vi "iWorx - Water Quality Lab.vi"() -> ()   [LabVIEW 2012]
uses:
  <vilib>/Utility/miscctls.llb/LVRangeTypeDef.ctl
  <vilib>/DAQmx/read.llb/DAQmx Read (Analog 1D Wfm NChan 1Samp).vi
  <vilib>/DAQmx/create/channels.llb/DAQmx Create Channel (AI-Voltage-Basic).vi
  <vilib>/DAQmx/miscellaneous.llb/DAQmx Fill In Error Info.vi
panel:
  in  "Mode":u16(ring) items=["Dissolved Oxygen", "pH", "Conductivity", "Turbidity"]
  in  "Set Up":bool
  out "Offset":dbl=-47.39336492890996
  out "Slope":dbl=47.39336492890995
  in  "Set SP2":bool
  in  "Set SP1":bool
  in  "Calibration Data":T1={"SP1 Voltage"=3.11, "SP2 Voltage"=1.0, "SP1 Value"=100.0, "SP2 Value"=0.0} {"SP2 Voltage" format="%#_g V"; "SP1 Voltage" format="%#_g V"}
  in  "Pause Button":bool
  in  "Snapshot":bool
  out "Processed Signal":dbl(knob) caption="Oxygen Content" scale=0.0..100.0
  in  "stop":bool
  out "Waveform Chart":waveform(dbl)(graph)
  in  "Sample Timing":u16(ring)=200 items=["20Hz"=50, "5 Hz"=200, "2 Hz"=500, "1 Hz"=1000, ".5 Hz"=2000, ".2 Hz"=5000]
  in  "Clear Chart":bool
  in  "Open Log":bool
  in  "Autoscale Y":bool
  out "Raw Signal":dbl(knob) scale=-5.0..5.0
  # "Water Quality Lab"
  # "Sensor Input (Ch 1)"
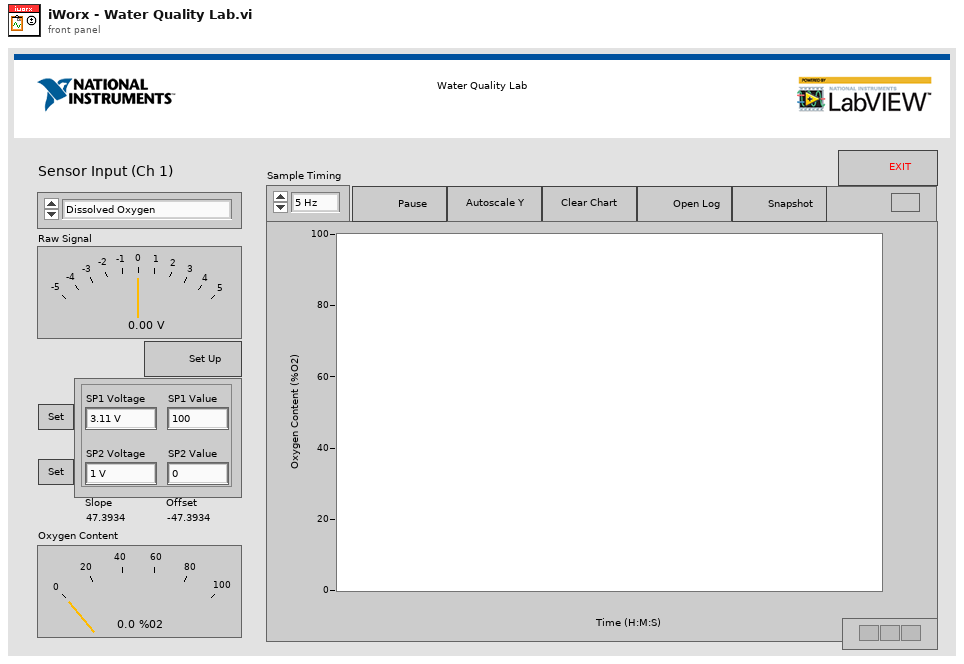
[diagram p1: front panel]
types:
  T1 = cluster{"SP1 Voltage":dbl, "SP2 Voltage":dbl, "SP1 Value":dbl, "SP2 Value":dbl}
  T2 = typedef "LVRangeTypeDef.ctl" = cluster{"Minimum":dbl, "Maximum":dbl, "Increment":dbl, "Minor Increment":dbl, "Start":dbl}
  T3 = cluster{"Name":string, "Format String":string, "Y Scale Name":string, "Scale.Range":T2, "Calibration Data":cluster{"SP1 Voltage":dbl, "SP2 Voltage":dbl, "SP1 Value":dbl, "SP2 Value":dbl}}[]
  T4 = cluster{"Name":string, "Format String":string, "Y Scale Name":string, "Scale.Range":T2, "Calibration Data":cluster{"SP1 Voltage":dbl, "SP2 Voltage":dbl, "SP1 Value":dbl, "SP2 Value":dbl}}
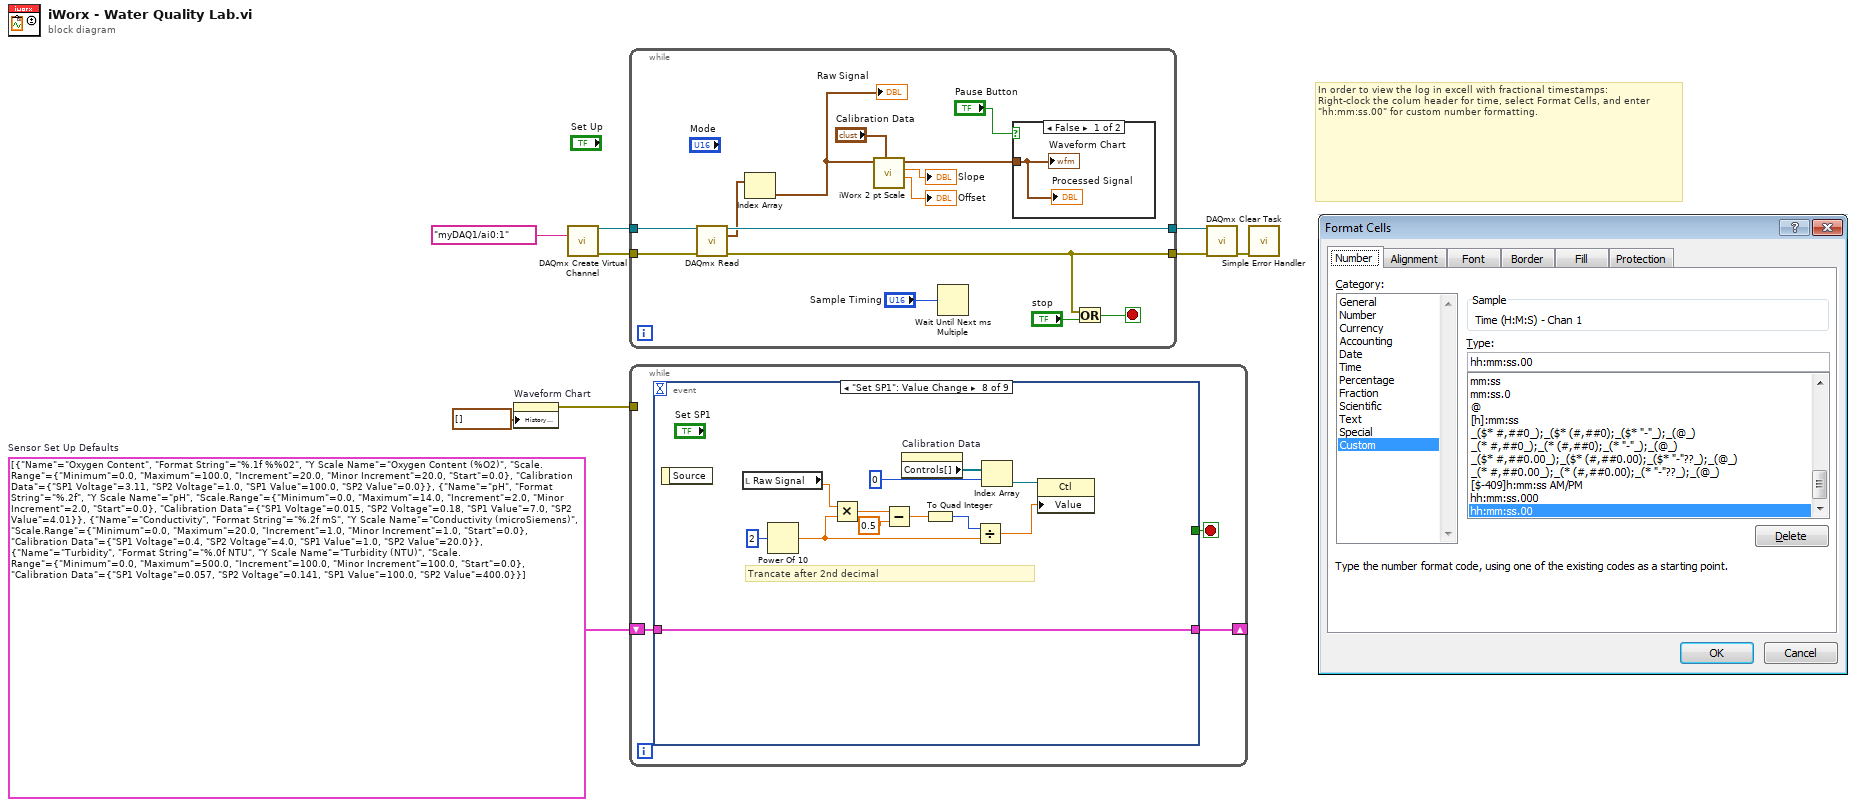
[diagram p0: block diagram]
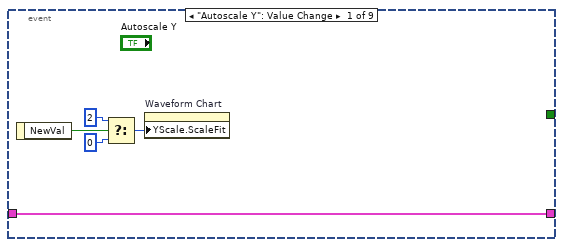
[diagram p2: hidden frame]
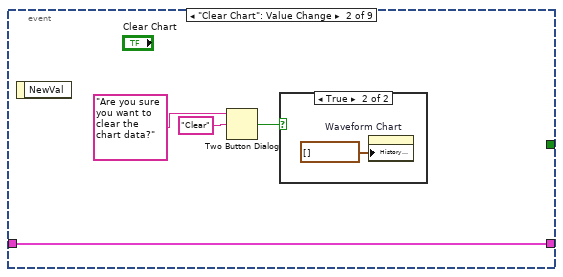
[diagram p3: hidden frame]
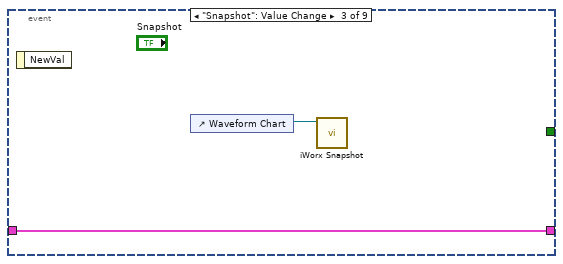
[diagram p5: hidden frame]
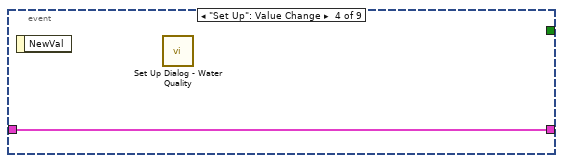
[diagram p6: hidden frame]
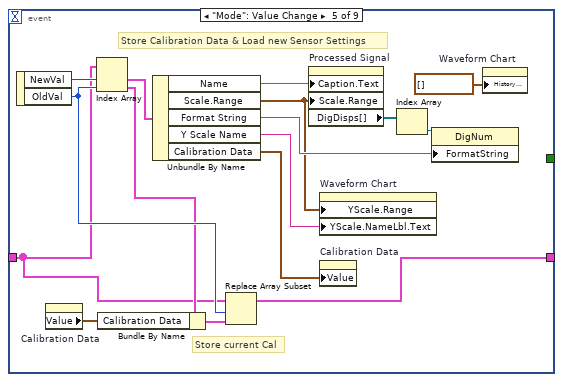
[diagram p7: hidden frame]
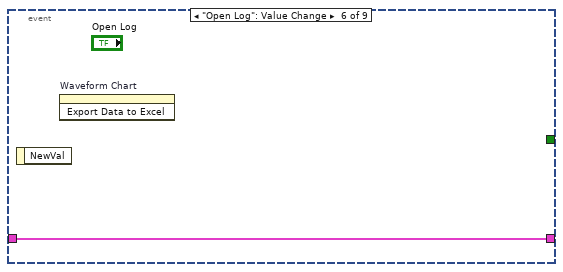
[diagram p8: hidden frame]
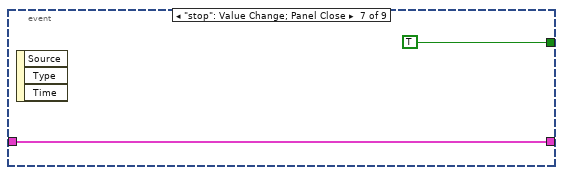
[diagram p9: hidden frame]
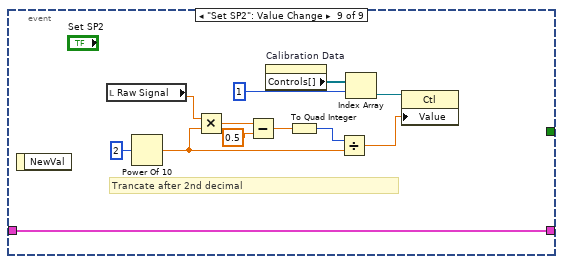
[diagram p10: hidden frame]
diagram:
  w1 = T3 [{"Name"="Oxygen Content", "Format String"="%.1f %%02", "Y Scale Name"="Oxygen Content (%O2)", "Scale.Range"={"Minimum"=0.0, "Maximum"=100.0, "Increment"=20.0, "Minor Increment"=20.0, "Start"=0.0}, "Calibration Data"={"SP1 Voltage"=3.11, "SP2 Voltage"=1.0, "SP1 Value"=100.0, "SP2 Value"=0.0}}, {"Name"="pH", "Format String"="%.2f", "Y Scale Name"="pH", "Scale.Range"={"Minimum"=0.0, "Maximum"=14.0, "Increment"=2.0, "Minor Increment"=2.0, "Start"=0.0}, "Calibration Data"={"SP1 Voltage"=0.015, "SP2 Voltage"=0.18, "SP1 Value"=7.0, "SP2 Value"=4.01}}, {"Name"="Conductivity", "Format String"="%.2f mS", "Y Scale Name"="Conductivity (microSiemens)", "Scale.Range"={"Minimum"=0.0, "Maximum"=20.0, "Increment"=1.0, "Minor Increment"=1.0, "Start"=0.0}, "Calibration Data"={"SP1 Voltage"=0.4, "SP2 Voltage"=4.0, "SP1 Value"=1.0, "SP2 Value"=20.0}}, {"Name"="Turbidity", "Format String"="%.0f NTU", "Y Scale Name"="Turbidity (NTU)", "Scale.Range"={"Minimum"=0.0, "Maximum"=500.0, "Increment"=100.0, "Minor Increment"=100.0, "Start"=0.0}, "Calibration Data"={"SP1 Voltage"=0.057, "SP2 Voltage"=0.141, "SP1 Value"=100.0, "SP2 Value"=400.0}}]  # Sensor Set Up Defaults
  # "In order to view the log in excell with fractional timestamps: \nRight-clock the colum header for time, select Format Cells, and enter \"hh:mm:ss.00\" for custom number formatting."
  n1 = property on="Waveform Chart" class="WFChart (strict)"("History Data"=waveform(dbl)[] []) -> (error out=w4:errorcluster)  [unwired: 2 in, 1 out]
  n2 = call-poly <vilib>:"DAQmx Create Virtual Channel.vi"("physical channels"=tag "myDAQ1/ai0:1") -> ("task out"=w6:refnum<k21>, "error out"=w5:errorcluster)  [unwired: 13 in]
  n3 = while {
    tunnel: w6 -> [w21]
    tunnel: [w20] -> w9
    tunnel: w5 -> [w19]
    tunnel: [w17] -> w8
    stop <- w18 stop-if-true
    n4 = call-poly <vilib>:"DAQmx Read.vi"("task/channels in"=w21, "error in"=w19) -> ("task out"=w20:refnum<k21>, "data"=w15:waveform(dbl)[], "error out"=w17:errorcluster)  [unwired: 11 in]
    n5 = Index Array(array=w15) -> (element=w13:waveform(dbl))  [unwired: 1 in]
    "Raw Signal" <- w13
    n6 = call "iWorx 2 pt Scale.vi"("Calibration Data"="Calibration Data", "Raw Waveform"=w13) -> ("Offset"=→"Offset":dbl, "Slope"=→"Slope":dbl, "Scaled Value"=w14:waveform(dbl))  [unwired: 7 in]
    n7 = Wait Until Next ms Multiple(millisecond multiple="Sample Timing") -> ()  [unwired: 1 out]
    n8 = case shown="False" "Pause Button" {
      tunnel: w14 -> [w24 _]
      frame False {
        "Waveform Chart" <- w24
        "Processed Signal" <- w24
      }
      frame True {
      }
    }
    n9 = Or(x=w17, y="stop") -> (x .or. y?=w18:bool)
  }
  n10 = while {
    tunnel: w4 -> [_]
    shift-right: [w25] -> _
    shift-left: w1 -> [w26]
    stop <- w27 stop-if-true
    n11 = event shown="[7] \"Set SP1\": Value Change" {
      selector: _ -> [_ _ _ _ _ _ _ _ _]
      dyn-events: _ -> [_ _ _ _ _ _ _ _ _]
      timeout: _ -> [_ _ _ _ _ _ _ _ _]
      tunnel: [_ _ _ _ _ _ TRUE _ _] -> w27
      tunnel: w26 -> [w28 w33 w38 w40 w41 w57 w58 w60 w72]
      tunnel: [w28 w33 w38 w40 w46 w57 w58 w60 w72] -> w25
      event "Autoscale Y": Value Change {
        n12 = event-data() -> ("NewVal"=w30:bool)  [unwired: 1 in]
        n13 = Select(t=u8 2 ("Y Scale.Scale Fit"), s=w30, f=u8 0 ("Y Scale.Scale Fit")) -> (s? t:f=w29:u8)
        n14 = property on="Waveform Chart" class="WFChart (strict)"("YScale.ScaleFit"=w29) -> ()  [unwired: 2 in, 2 out]
      }
      event "Clear Chart": Value Change {
        n15 = event-data() -> ()  [unwired: 1 in, 1 out]
        n16 = Two Button Dialog(message="Are you sure you want to clear the chart data?", 2:"Clear" ("T button name (\"OK\")")) -> (T button?=w35:bool)  [unwired: 1 in]
        n17 = case shown="True" w35 {
          frame False {
          }
          frame True {
            n18 = property on="Waveform Chart" class="WFChart (strict)"("History Data"=waveform(dbl)[] []) -> ()  [unwired: 2 in, 2 out]
          }
        }
      }
      event "Snapshot": Value Change {
        n19 = event-data() -> ()  [unwired: 1 in, 1 out]
        n20 = control-ref of="Waveform Chart"() -> (w39:refnum<vi>)
        n21 = call "iWorx Snapshot.vi"("WaveformChart in"=w39) -> ()  [unwired: 10 in, 1 out]
      }
      event "Set Up": Value Change {
        n22 = event-data() -> ()  [unwired: 1 in, 1 out]
        n23 = call "Set Up Dialog - Water Quality.vi"() -> ()  [unwired: 12 in]
      }
      event "Mode": Value Change {
        # "Store current Cal"
        # "Store Calibration Data & Load new Sensor Settings"
        n24 = event-data() -> ("NewVal"=w49:u16, "OldVal"=w47:u16)  [unwired: 1 in]
        n25 = property on="Calibration Data" class="Clust (strict)"() -> ("Value"=w45:T1)  [unwired: 2 in, 2 out]
        n26 = Index Array(array=w41, index #1=w49, index #2=w47) -> (element #1=w48:T4, element #2=w42:T4)
        n27 = Bundle By Name(cluster=w42, "Calibration Data"=w45) -> (w44:T4)
        n28 = Unbundle By Name(w48) -> ("Name"=w54:string, "Scale.Range"=w52:T2, "Format String"=w53:string, "Y Scale Name"=w51:string, "Calibration Data"=w50:T1)
        n29 = Replace Array Subset(array=w41, new element=w44, index=w47) -> (w46:T3)
        n30 = property on="Processed Signal" class="Knob (strict)"("Caption.Text"=w54, "Scale.Range"=w52) -> ("DigDisps[]"=w55:refnum<vi>[])  [unwired: 2 in, 2 out]
        n31 = property on="Waveform Chart" class="WFChart (strict)"("YScale.Range"=w52, "YScale.NameLbl.Text"=w51) -> ()  [unwired: 2 in, 2 out]
        n32 = property on="Calibration Data" class="Clust (strict)"("Value"=w50) -> ()  [unwired: 2 in, 2 out]
        n33 = Index Array(array=w55) -> (element=w56:refnum<vi>)  [unwired: 1 in]
        n34 = property class="DigNum"(reference=w56, "FormatString"=w53) -> ()  [unwired: 1 in, 2 out]
        n35 = property on="Waveform Chart" class="WFChart (strict)"("History Data"=waveform(dbl)[] []) -> ()  [unwired: 2 in, 2 out]
      }
      event "Open Log": Value Change {
        n36 = event-data() -> ()  [unwired: 1 in, 1 out]
        n37 = invoke on="Waveform Chart" class="WFChart (strict)" method="Export Data to Excel"() -> ()  [unwired: 3 in, 3 out]
      }
      event "stop": Value Change; Panel Close {
        n38 = event-data() -> ()  [unwired: 1 in, 3 out]
      }
      event "Set SP1": Value Change {
        # "Trancate after 2nd decimal"
        n39 = event-data() -> ()  [unwired: 1 in, 1 out]
        n40 = local read "Raw Signal"() -> (w61:dbl)
        n41 = Power Of 10(x=2) -> (10^x=w68:dbl)
        n42 = Multiply(x=w61, y=w68) -> (x*y=w66:dbl)
        n43 = Subtract(x=w66, y=0.5) -> (x-y=w65:dbl)
        n44 = property on="Calibration Data" class="Clust (strict)"() -> ("Controls[]"=w71:refnum<vi>[])  [unwired: 2 in, 2 out]
        n45 = To Quad Integer(1:w65) -> (0:w67:i64)
        n46 = Divide(x=w67, y=w68) -> (x/y=w63:dbl)
        n47 = Index Array(array=w71, index=0) -> (element=w70:refnum<vi>)
        n48 = property class="Ctl"(reference=w70, "Value"=w63) -> ()  [unwired: 1 in, 2 out]
      }
      event "Set SP2": Value Change {
        # "Trancate after 2nd decimal"
        n49 = event-data() -> ()  [unwired: 1 in, 1 out]
        n50 = local read "Raw Signal"() -> (w73:dbl)
        n51 = Power Of 10(x=2) -> (10^x=w80:dbl)
        n52 = Multiply(x=w73, y=w80) -> (x*y=w78:dbl)
        n53 = Subtract(x=w78, y=0.5) -> (x-y=w77:dbl)
        n54 = property on="Calibration Data" class="Clust (strict)"() -> ("Controls[]"=w83:refnum<vi>[])  [unwired: 2 in, 2 out]
        n55 = To Quad Integer(1:w77) -> (0:w79:i64)
        n56 = Divide(x=w79, y=w80) -> (x/y=w75:dbl)
        n57 = Index Array(array=w83, index=1) -> (element=w82:refnum<vi>)
        n58 = property class="Ctl"(reference=w82, "Value"=w75) -> ()  [unwired: 1 in, 2 out]
      }
    }
  }
  n59 = call <vilib>:"DAQmx Clear Task.vi"("task in"=w9, "error in"=w8) -> ("error out"=w3:errorcluster)  [unwired: 13 in]
  n60 = call <vilib>:"Simple Error Handler.vi"("error in (no error)"=w3) -> ()  [unwired: 4 in, 5 out]
